vi "Arm Activation.vi"() -> ()   [LabVIEW 2014]
panel:
  in  "Enum":enum16{"Up", "Down", "Manual Disable"}(ring)
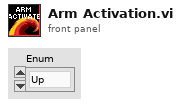
[diagram p1: front panel]
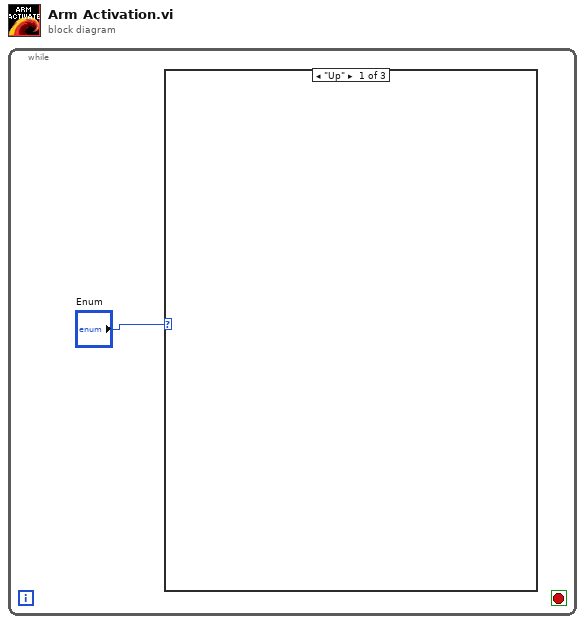
[diagram p0: block diagram]
diagram:
  n1 = while {
    stop <- _ stop-if-true
    n2 = case shown="\"Up\"" "Enum" {
      frame "Up" {
      }
      frame "Down" {
      }
      frame "Manual Disable", Default {
      }
    }
  }
